vi "Effects Player.vi"(11 "Command Queue":refnum<queue>) -> ()   [LabVIEW 2019, in "Sound.lvlib"]
doc: "A single channel sound effects player. Issue commands to it via the command queue. Note that if a sound effect is already playing, new sound effects will not be played until completion of playback. It is possible to stop the sound effect output if needed."
uses:
  Sound.lvlib
  Music Player Command Message.ctl
  Music Player Command.ctl
  <vilib>/sound2/lvsound2.llb/Sound Output Task ID.ctl
  Effects Player State.ctl
  <vilib>/sound2/lvsound2.llb/Sampling Mode.ctl
  <vilib>/sound2/lvsound2.llb/Sound Data Format.ctl
  <vilib>/sound2/lvsound2.llb/Sound Output Write (I16).vi
  _LabVIEW Audio Codecs/LabVIEW Audio Codecs.lvlib
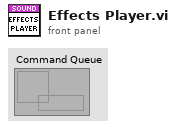
[diagram p1: front panel]
types:
  T1 = typedef "Sound.lvlib/Effects Player State.ctl" = enum16{"Load Effects", "Check Command", "Play", "Stop", "Shutdown"}
  T2 = typedef "Sound Output Task ID.ctl" = u32
  T3 = typedef "Sound Data Format.ctl" = cluster{"sample rate (S/s)":dbl, "number of channels":i32, "bits per sample":i32}
  T4 = typedef "Sound.lvlib/Music Player Command Message.ctl" = cluster{"Command":T5, "Data":variant}
  T5 = typedef "Sound.lvlib/Music Player Command.ctl" = enum16{"Enable", "Play", "Play Random", "Stop", "Shutdown"}
  T6 = typedef "Sampling Mode.ctl" = i32
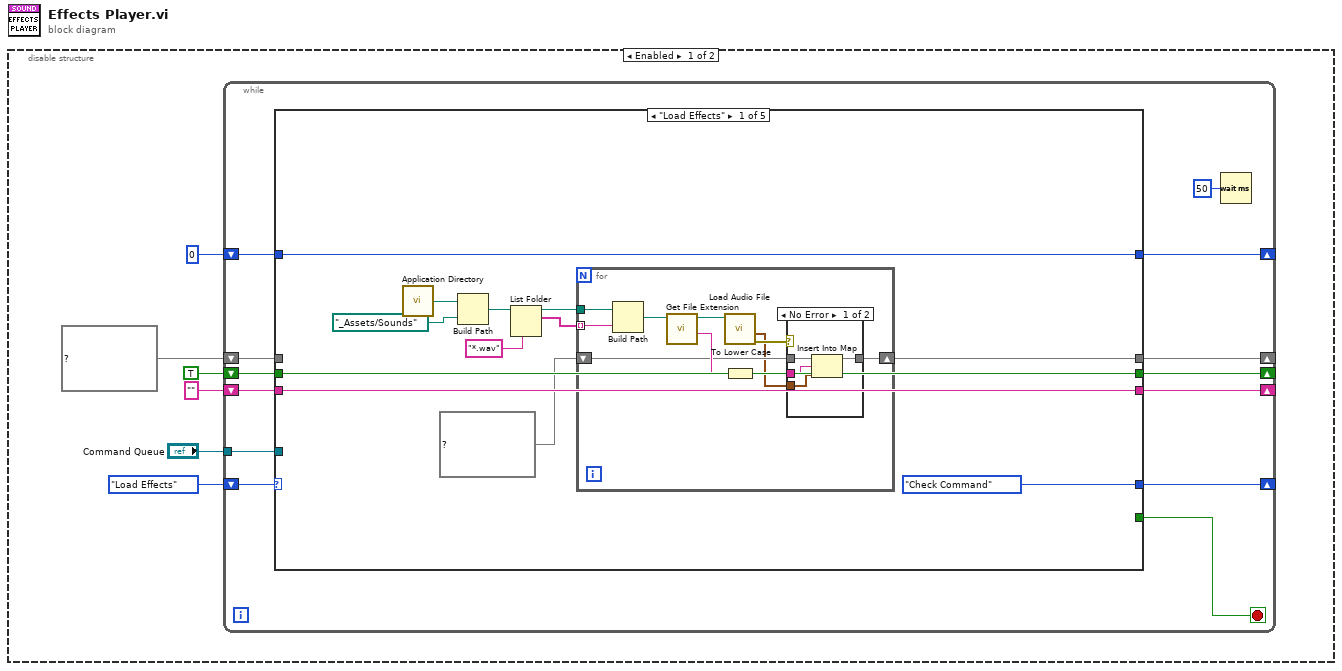
[diagram p0: block diagram]
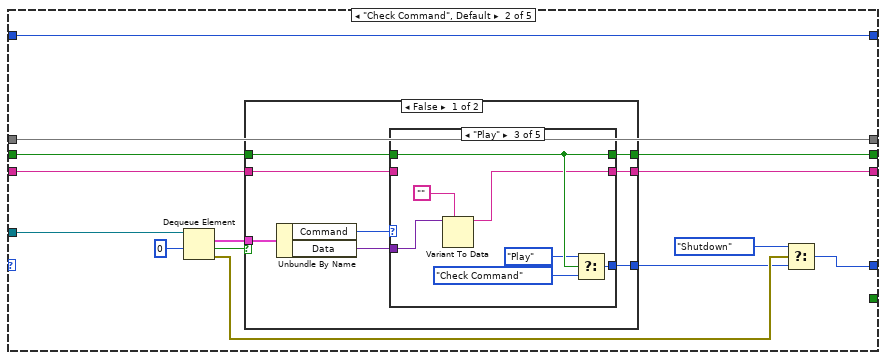
[diagram p3: hidden frame]
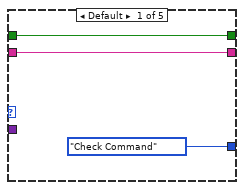
[diagram p4: hidden frame]
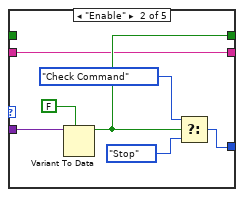
[diagram p5: hidden frame]
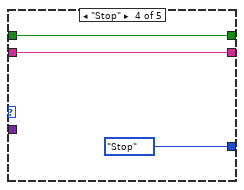
[diagram p6: hidden frame]
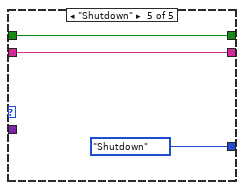
[diagram p7: hidden frame]
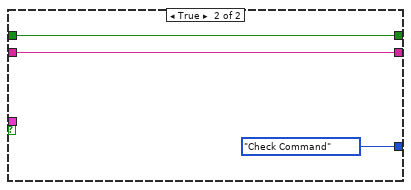
[diagram p8: hidden frame]
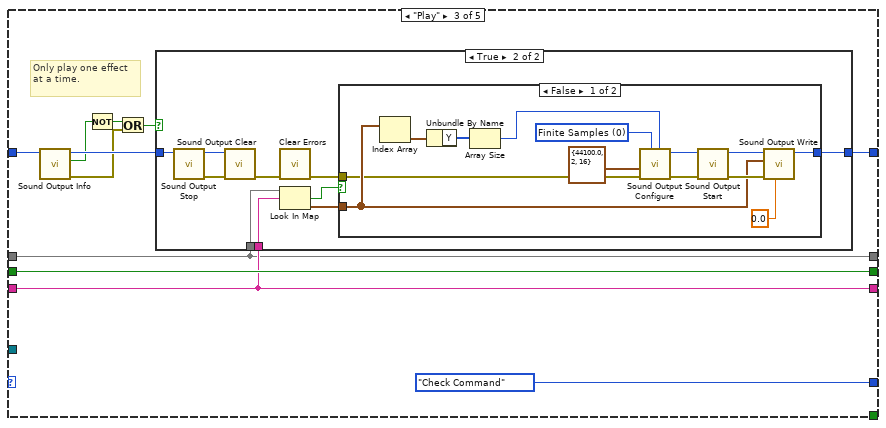
[diagram p9: hidden frame]
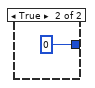
[diagram p11: hidden frame]
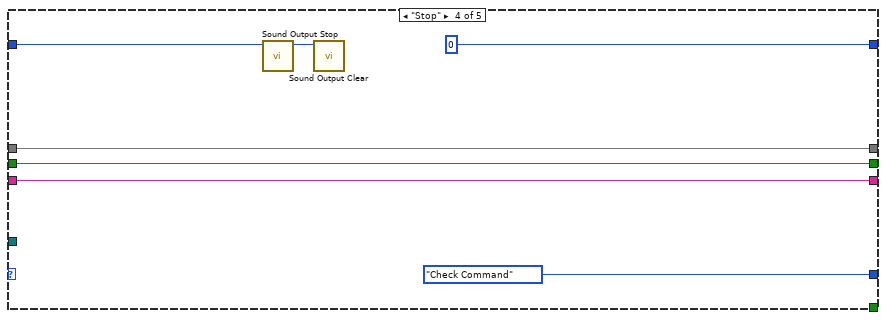
[diagram p12: hidden frame]
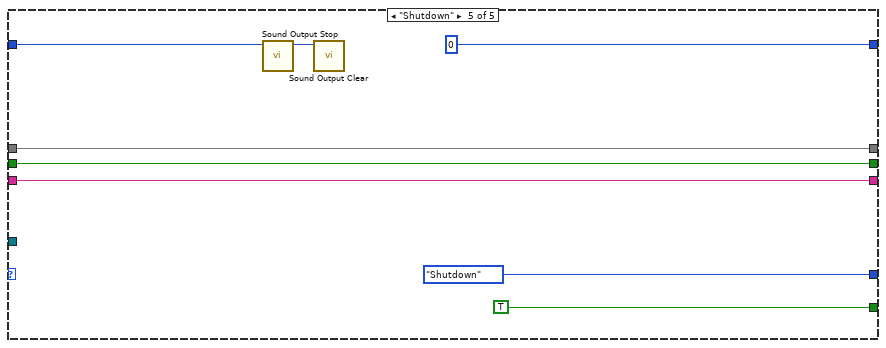
[diagram p13: hidden frame]
diagram:
  n1 = disable-structure shown="Enabled" {
    frame Enabled {
      n2 = while {
        shift-right: [w19] -> _
        shift-left: T2 0 ("task ID out") -> [w18]
        shift-right: [w16] -> _
        shift-left: Effects_Player_State."Load Effects" ("Effects Player State") -> [w17]
        tunnel: "Command Queue" -> [w14]
        shift-right: [w13] -> _
        shift-left: TRUE -> [w12]
        shift-right: [w11] -> _
        shift-left: "" -> [w10]
        shift-right: [w8] -> _
        shift-left: map{string, waveform(i16)[]} {} ("map") -> [w7]
        stop <- w15 stop-if-true
        n3 = case shown="\"Load Effects\"" w17 {
          tunnel: [w31 w60 w105 T2 0 ("task ID out") T2 0 ("task ID out")] -> w19
          tunnel: w18 -> [w31 w60 w100 w137 w145]
          tunnel: [Effects_Player_State."Check Command" ("Effects Player State") w48 Effects_Player_State."Check Command" Effects_Player_State."Check Command" ("f") Effects_Player_State."Shutdown" ("f")] -> w16
          tunnel: [_ _ _ _ TRUE] -> w15
          tunnel: w14 -> [_ w59 _ _ _]
          tunnel: [w30 w55 w103 w133 w141] -> w13
          tunnel: w12 -> [w30 w54 w103 w133 w141]
          tunnel: [w29 w53 w102 w132 w140] -> w11
          tunnel: w10 -> [w29 w52 w102 w132 w140]
          tunnel: [w21 w51 w101 w131 w139] -> w8
          tunnel: w7 -> [_ w51 w101 w131 w139]
          frame "Load Effects" {
            n4 = call <vilib>:"Application Directory.vi"() -> ("Application Directory"=w24:path)
            n5 = Build Path(base path=w24, name or relative path=path "_Assets/Sounds" ("path")) -> (appended path=w22:path)
            n6 = List Folder(path=w22, pattern="*.wav") -> (path out=w26:path, filenames=w25:string[])  [unwired: 2 in, 2 out]
            n7 = for {
              tunnel: w26 -> [w41]
              tunnel: w25 -> [w40] mode=indexing
              shift-right: [w33] -> w21
              shift-left: map{string, waveform(i16)[]} {} ("map") -> [w34]
              n8 = Build Path(base path=w41, name or relative path=w40) -> (appended path=w39:path)
              n9 = call <vilib>:"Get File Extension.vi"("file"=w39) -> ("filename without extension"=w37:string, "dup file"=w38:path)  [unwired: 6 in, 3 out]
              n10 = call "Load Audio File.vi"("Path"=w38) -> ("error out"=w36:errorcluster, "Data"=w32:waveform(i16)[])  [unwired: 6 in, 3 out]
              n11 = To Lower Case(string=w37) -> (all lower case string=w35:string)
              n12 = case shown="No Error" w36 {
                tunnel: w35 -> [w45 _]
                tunnel: w34 -> [w44 w46]
                tunnel: [w43 w46] -> w33
                tunnel: w32 -> [w42 _]
                frame No Error {
                  n13 = Insert Into Map(map in=w44, key=w45, value=w42) -> (map out=w43:map{string, waveform(i16)[]})  [unwired: 2 out]
                }
                frame Error {
                }
              }
            }
          }
          frame "Check Command", Default {
            n14 = Dequeue Element(queue=w59, timeout in ms (-1)=0) -> (element=w57:T4, timed out?=w56:bool, error out=w50:errorcluster)  [unwired: 1 in, 1 out]
            n15 = case shown="False" w56 {
              tunnel: w57 -> [w68 _]
              tunnel: [w63 Effects_Player_State."Check Command"] -> w49
              tunnel: [w65 w93] -> w55
              tunnel: w54 -> [w64 w93]
              tunnel: [w62 w92] -> w53
              tunnel: w52 -> [w61 w92]
              frame False {
                n16 = Unbundle By Name(w68) -> ("Command"=w67:T5, "Data"=w66:variant)
                n17 = case shown="\"Play\"" w67 {
                  tunnel: w66 -> [_ w78 w81 _ _]
                  tunnel: [w71 w76 w85 w88 w90] -> w65
                  tunnel: w64 -> [w71 _ w85 w88 w90]
                  tunnel: [Effects_Player_State."Check Command" w75 w84 Effects_Player_State."Stop" ("f") Effects_Player_State."Shutdown" ("f")] -> w63
                  tunnel: [w69 w72 w79 w87 w89] -> w62
                  tunnel: w61 -> [w69 w72 _ w87 w89]
                  frame Default {
                  }
                  frame "Enable" {
                    n18 = Variant To Data(type=FALSE, Variant=w78) -> (data=w76:bool)  [unwired: 1 in, 1 out]
                    n19 = Select(t=Effects_Player_State."Check Command", s=w76, f=Effects_Player_State."Stop") -> (s? t:f=w75:T1)
                  }
                  frame "Play" {
                    n20 = Variant To Data(type="", Variant=w81) -> (data=w79:string)  [unwired: 1 in, 1 out]
                    n21 = Select(t=Effects_Player_State."Play", s=w85, f=Effects_Player_State."Check Command") -> (s? t:f=w84:T1)
                  }
                  frame "Stop" {
                  }
                  frame "Shutdown" {
                  }
                }
              }
              frame True {
              }
            }
            n22 = Select(t=Effects_Player_State."Shutdown", s=w50, f=w49) -> (s? t:f=w48:T1)
          }
          frame "Play" {
            # "Only play one effect at a time."
            n23 = call <vilib>:"Sound Output Info.vi"("task ID"=w100) -> ("error out"=w97:errorcluster, "is playing?"=w98:bool, "task ID out"=w99:T2)  [unwired: 7 in, 1 out]
            n24 = Not(x=w98) -> (.not. x?=w95:bool)
            n25 = Or(x=w95, y=w97) -> (x .or. y?=w96:bool)
            n26 = case shown="True" w96 {
              tunnel: [w106 w116] -> w105
              tunnel: w99 -> [w106 w114]
              tunnel: w102 -> [_ w111]
              tunnel: w101 -> [_ w107]
              frame False {
              }
              frame True {
                n27 = call <vilib>:"Sound Output Stop.vi"("task ID"=w114) -> ("error out"=w113:errorcluster, "task ID out"=w115:T2)  [unwired: 9 in]
                n28 = call <vilib>:"Sound Output Clear.vi"("error in (no error)"=w113, "task ID"=w115) -> ("error out"=w112:errorcluster)  [unwired: 9 in]
                n29 = call <vilib>:"Clear Errors.vi"("error in (no error)"=w112) -> ("error out"=w109:errorcluster)  [unwired: 5 in, 1 out]
                n30 = Look In Map(map=w107, key=w111) -> (key not found?=w108:bool, value=w110:waveform(i16)[])  [unwired: 1 in]
                n31 = case shown="False" w108 {
                  tunnel: [w122 T2 0 ("task ID out")] -> w116
                  tunnel: w110 -> [w121 _]
                  tunnel: w109 -> [w117 _]
                  frame False {
                    w129 = T6 0 items=["Finite Samples", "Continuous Samples"] ("sample mode")
                    n32 = Index Array(array=w121) -> (element=w120:waveform(i16))  [unwired: 1 in]
                    n33 = Unbundle By Name(w120) -> ("Y"=w119:i16[])
                    n34 = Array Size(array=w119) -> (size(s)=w118:i32)
                    n35 = call <vilib>:"Sound Output Configure.vi"("number of samples/ch"=w118, "sample mode"=w129, "error in (no error)"=w117, "sound format"=T3 {"sample rate (S/s)"=44100.0, "number of channels"=2, "bits per sample"=16}) -> ("error out"=w126:errorcluster, "task ID"=w127:T2)  [unwired: 6 in]
                    n36 = call <vilib>:"Sound Output Start.vi"("error in (no error)"=w126, "task ID"=w127) -> ("error out"=w125:errorcluster, "task ID out"=w124:T2)  [unwired: 8 in]
                    n37 = call-poly <vilib>:"Sound Output Write.vi"("timeout (sec)"=0.0, "error in (no error)"=w125, "data"=w121, "task ID"=w124) -> ("task ID out"=w122:T2)  [unwired: 6 in, 1 out]
                  }
                  frame True {
                  }
                }
              }
            }
          }
          frame "Stop" {
            n38 = call <vilib>:"Sound Output Stop.vi"("task ID"=w137) -> ("task ID out"=w136:T2)  [unwired: 9 in, 1 out]
            n39 = call <vilib>:"Sound Output Clear.vi"("task ID"=w136) -> ()  [unwired: 10 in, 1 out]
          }
          frame "Shutdown" {
            n40 = call <vilib>:"Sound Output Stop.vi"("task ID"=w145) -> ("task ID out"=w144:T2)  [unwired: 9 in, 1 out]
            n41 = call <vilib>:"Sound Output Clear.vi"("task ID"=w144) -> ()  [unwired: 10 in, 1 out]
          }
        }
        n42 = Wait (ms)(milliseconds to wait=u32 50) -> ()  [unwired: 1 out]
      }
    }
    frame Disabled {
    }
  }
